vi "Dequeue.vi"(8 "error in (no error)":errorcluster, 10 "timeout in ms (100)":i32=100, 11 "queue":refnum<queue>) -> (0 "error out":errorcluster, 1 "Value":string, 2 "Command":string, 3 "queue out":refnum<queue>)   [LabVIEW 2014, in "Raspberry Pi Compatible Compiler for LabVIEW.lvlib"]
uses:
  Raspberry Pi Compatible Compiler for LabVIEW.lvlib
  Custom Controls/Queue Message.ctl
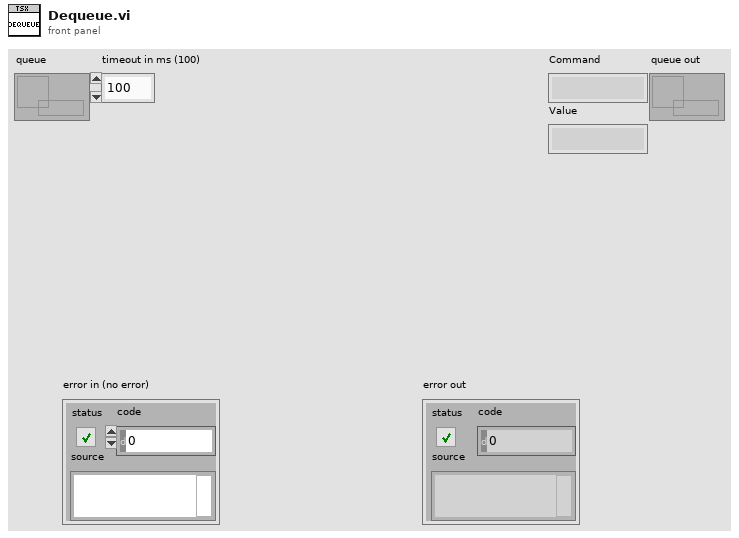
[diagram p1: front panel]
types:
  T1 = typedef "Raspberry Pi Compatible Compiler for LabVIEW.lvlib/Queue Message.ctl" = cluster{"Command":string, "Value":string}
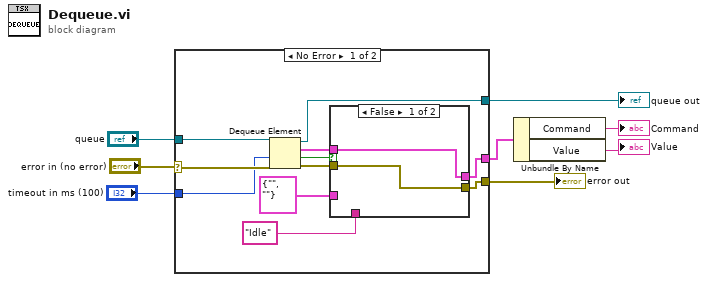
[diagram p0: block diagram]
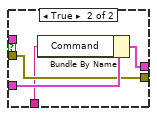
[diagram p2: hidden frame]
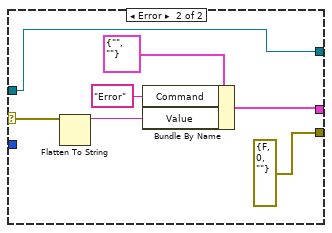
[diagram p3: hidden frame]
diagram:
  n1 = case shown="No Error" "error in (no error)" {
    selector: "error in (no error)" -> [w15 w32]
    tunnel: [w12 errorcluster {"status"=FALSE, "code"=0, "source"=""} ("error IO")] -> w7
    tunnel: [w13 w27] -> w6
    tunnel: "queue" -> [w19 w26]
    tunnel: [w18 w26] -> w2
    tunnel: "timeout in ms (100)" -> [w9 _]
    frame No Error {
      n2 = Dequeue Element(queue=w19, timeout in ms (-1)=w9, error in (no error)=w15) -> (queue out=w18:refnum<queue>, element=w10:T1, timed out?=w17:bool, error out=w16:errorcluster)
      n3 = case shown="False" w17 {
        tunnel: w16 -> [w20 w23]
        tunnel: T1 {"Command"="", "Value"=""} ("Message") -> [_ w25]
        tunnel: [w21 w24] -> w13
        tunnel: [w20 w23] -> w12
        tunnel: "Idle" ("Command") -> [_ w22]
        tunnel: w10 -> [w21 _]
        frame False {
        }
        frame True {
          n4 = Bundle By Name(cluster=w25, "Command"=w22) -> (w24:T1)
        }
      }
    }
    frame Error {
      n5 = Flatten To String(anything=w32) -> (data string=w29:string)  [unwired: 1 in, 4 out]
      n6 = Bundle By Name(cluster=T1 {"Command"="", "Value"=""} ("Message"), "Command"="Error", "Value"=w29) -> (w27:T1)
    }
  }
  "error out" <- w7
  "queue out" <- w2
  n7 = Unbundle By Name(w6) -> ("Command"=→"Command":string, "Value"=→"Value":string)
